vi "fgt get sensor Air Bubble Flag.vi"(8 "error in (no error)":errorcluster, 11 "sensorIndex":u32) -> (0 "error out":errorcluster, 3 "air bubble?":bool)   [LabVIEW 2016, in "fgt_SDK.lvlib"]
doc: "Read the flag indicating whether the flow rate sensor detects an air bubble. Only available on Flow Unit sensor ranges M+ and L+."
uses:
  fgt_SDK.lvlib
  dlls/fgt_SDK_32.dll
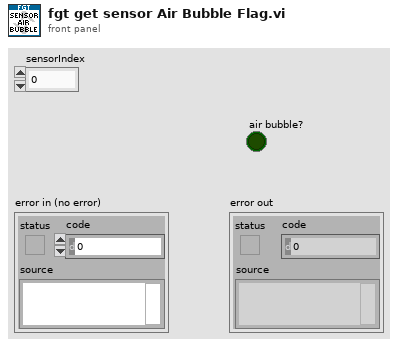
[diagram p1: front panel]
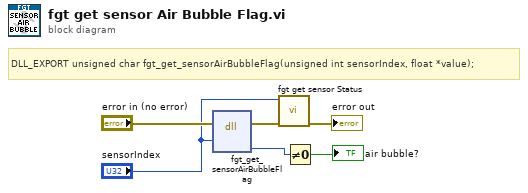
[diagram p0: block diagram]
diagram:
  # "DLL_EXPORT unsigned char fgt_get_sensorAirBubbleFlag(unsigned int sensorIndex, float *value);"
  n1 = dll-call lib="C:/projects/SDK/fgt-sdk-labview/dlls/fgt_SDK_*.*" fn="fgt_get_sensorAirBubbleFlag"(error in="error in (no error)", "sensorIndex"="sensorIndex") -> (error out=w5:errorcluster, "value"=w2:u8)  [unwired: 5 in, 1 out]
  n2 = call "fgt get sensor Status.vi"("error in (no error)"=w5, "pressureIndex"="sensorIndex") -> ("error out"=→"error out":errorcluster)  [unwired: 9 in]
  n3 = Not Equal To 0?(x=w2) -> (x != 0?=→"air bubble?":bool)
